vi "Tektronix TDS 200 1000 2000 Series Acquire Continuous Waveform.vi"() -> ()   [LabVIEW 2012]
doc: "This example shows how to use autosetup and acquire a waveform on a single channel."
uses:
  <instrlib>/Tektronix TDS 200 1000 2000 Series/Tektronix TDS 200 1000 2000 Series.lvlib
panel:
  in  "Source (0: Channel 1)":u16(ring) items=["Channel 1", "Channel 2", "Channel 3", "Channel 4", "Math", "Reference A", "Reference B", "Reference C", "Reference D"]
  in  "Serial Configuration":T1={"Baud Rate"=9600, "Parity"=0, "Stop Bits"=10, "Flow Control"=2} {"Flow Control" items=["None", "XON/XOFF", "RTS/CTS", "XON/XOFF & RTS/CTS", "DTR/DSR", "XON/XOFF & DTR/DSR"]; "Stop Bits" items=["1.0"=10, "1.5"=15, "2.0"=20]; "Parity" items=["None", "Odd", "Even", "Mark", "Space"]; "Baud Rate" items=["300"=300, "600"=600, "1200"=1200, "2400"=2400, "4800"=4800, "9600"=9600, "19200"=19200]}
  in  "stop":bool
  in  "Probe Attenuation (10.0)":dbl=10.0
  in  "Timeout (10000 ms)":u32=10000
  out "Waveform Data":waveform(dbl)(graph)
  in  "VISA resource name":refnum<visa-resource-name>
  # "(C) 2009-2014 National Instruments.  ALL RIGHTS RESERVED."
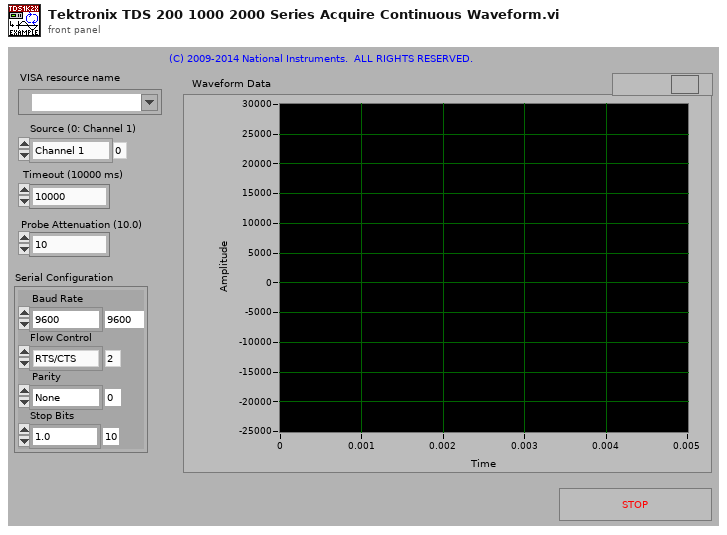
[diagram p1: front panel]
types:
  T1 = cluster{"Baud Rate":u32, "Parity":u16, "Stop Bits":u16, "Flow Control":u16}
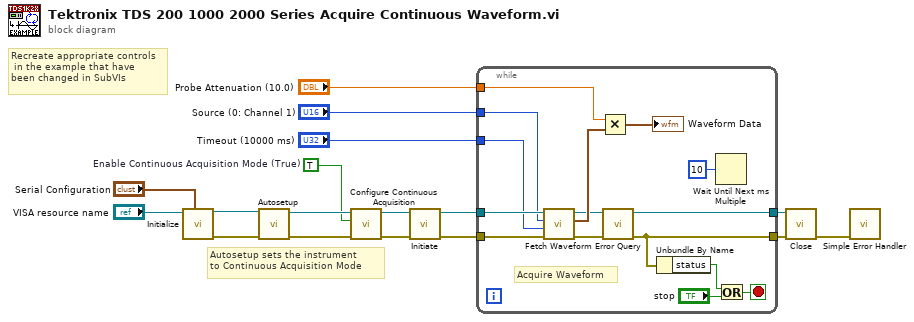
[diagram p0: block diagram]
diagram:
  w5 = TRUE  # Enable Continuous Acquisition Mode (True)
  # "Recreate appropriate controls\n in the example that have \nbeen changed in SubVIs"
  # "Autosetup sets the instrument\nto Continuous Acquisition Mode"
  n1 = call <instrlib>:"Initialize.vi"("Serial Configuration"="Serial Configuration", "VISA resource name"="VISA resource name") -> ("error out"=w12:errorcluster, "VISA resource name out"=w11:refnum<visa-resource-name>)  [unwired: 3 in, 5 out]
  n2 = call <instrlib>:"Autosetup.vi"("error in (no error)"=w12, "VISA resource name"=w11) -> ("error out"=w7:errorcluster, "VISA resource name out"=w6:refnum<visa-resource-name>)  [unwired: 8 out]
  n3 = call <instrlib>:"Configure Continuous Acquisition.vi"("error in (no error)"=w7, "Enable Continuous Acquisition Mode (True)"=w5, "VISA resource name"=w6) -> ("error out"=w4:errorcluster, "VISA resource name out"=w3:refnum<visa-resource-name>)  [unwired: 7 out]
  n4 = call <instrlib>:"Initiate.vi"("error in (no error)"=w4, "VISA resource name"=w3) -> ("error out"=w1:errorcluster, "VISA resource name out"=w2:refnum<visa-resource-name>)  [unwired: 8 out]
  n5 = while {
    tunnel: w2 -> [w32]
    tunnel: w1 -> [w31]
    tunnel: [w18] -> w16
    tunnel: [w21] -> w15
    tunnel: "Timeout (10000 ms)" -> [w30]
    tunnel: "Probe Attenuation (10.0)" -> [w29]
    tunnel: "Source (0: Channel 1)" -> [w22]
    stop <- w25 stop-if-true
    # "Acquire Waveform"
    n6 = call <instrlib>:"Fetch Waveform.vi"("error in (no error)"=w31, "Timeout (10000 ms)"=w30, "Source (0: Channel 1)"=w22, "VISA resource name"=w32) -> ("error out"=w20:errorcluster, "Waveform Data"=w28:waveform(dbl), "VISA resource name out"=w19:refnum<visa-resource-name>)  [unwired: 5 out]
    n7 = Multiply(x=w29, y=w28) -> (x*y=→"Waveform Data":waveform(dbl))
    n8 = call <instrlib>:"Error Query.vi"("error in (no error)"=w20, "VISA resource name"=w19) -> ("error out"=w21:errorcluster, "VISA resource name out"=w18:refnum<visa-resource-name>)  [unwired: 8 out]
    n9 = Unbundle By Name(w21) -> ("status"=w24:bool)
    n10 = Wait Until Next ms Multiple(millisecond multiple=u32 10) -> ()  [unwired: 1 out]
    n11 = Or(x=w24, y="stop") -> (x .or. y?=w25:bool)
  }
  n12 = call <instrlib>:"Close.vi"("error in (no error)"=w15, "VISA resource name"=w16) -> ("error out"=w17:errorcluster)  [unwired: 9 out]
  n13 = call <vilib>:"Simple Error Handler.vi"("error in (no error)"=w17) -> ()  [unwired: 1 in, 8 out]
